vi "resolve vi references.vi"(11 "remaining string":string) -> (2 "VI path":path, 3 "VI name":string)   [LabVIEW 2013, in "UI Reference configuration.lvclass"]
uses:
  UI Reference configuration.lvclass
  <vilib>/NI/Tag Bus Module Framework/root configuration/TBM configuration.lvclass
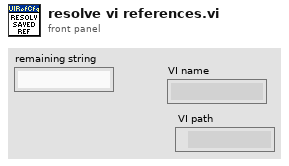
[diagram p1: front panel]
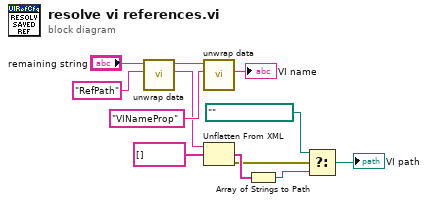
[diagram p0: block diagram]
diagram:
  n1 = call <vilib>:"unwrap data.vi"("identifier"="RefPath" ("additional identifier"), "data to unwrap"="remaining string") -> ("unwrapped data"=w8:string, "remaining string"=w11:string)  [unwired: 8 in]
  n2 = call <vilib>:"unwrap data.vi"("identifier"="VINameProp" ("additional identifier"), "data to unwrap"=w11) -> ("unwrapped data"=→"VI name":string)  [unwired: 8 in, 1 out]
  n3 = Unflatten From XML(xml string=w8, type=string[] [] ("array of strings")) -> (value=w6:string[], error out=w2:errorcluster)  [unwired: 1 in]
  n4 = Array of Strings to Path(0:w6) -> (2:w3:path)  [unwired: 1 in]
  n5 = Select(t=path "", s=w2, f=w3) -> (s? t:f=→"VI path":path)
